vi "shooter_flywheel_calc.vi"(0 "Close Shot":bool, 1 "Far Shot":bool, 2 "Custom Shot":bool, 3 "Close Voltage":dbl, 4 "Far Voltage":dbl, 5 "Custom Shot Voltage":dbl, 7 "Bus Voltage":dbl, 9 "Output Percent VBus":dbl) -> (14 "Voltage Output":dbl, 19 "Overloaded":bool)   [LabVIEW 2012]
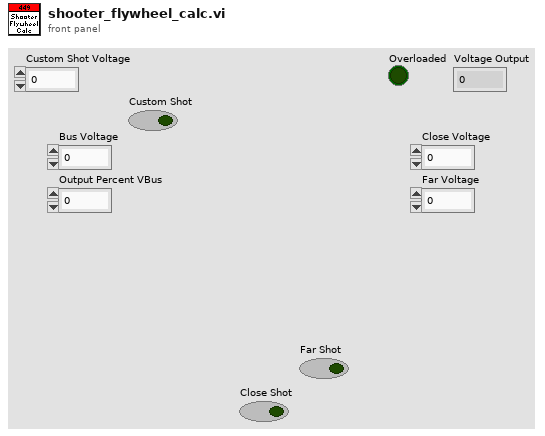
[diagram p1: front panel]
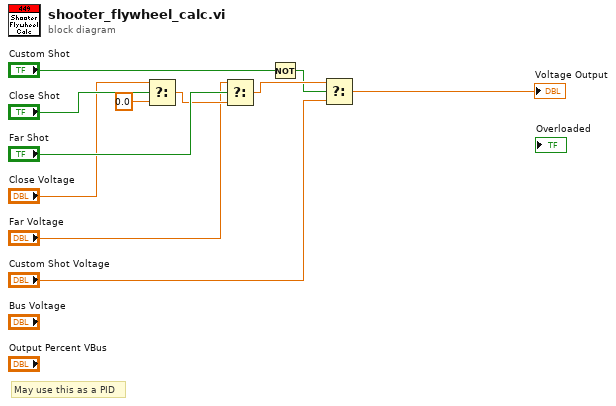
[diagram p0: block diagram]
diagram:
  # "May use this as a PID"
  n1 = Select(t="Close Voltage", s="Close Shot", f=0.0) -> (s? t:f=w7:dbl)
  n2 = Select(t="Far Voltage", s="Far Shot", f=w7) -> (s? t:f=w5:dbl)
  n3 = Not(x="Custom Shot") -> (.not. x?=w1:bool)
  n4 = Select(t=w5, s=w1, f="Custom Shot Voltage") -> (s? t:f=→"Voltage Output":dbl)
